vi "http 400 bad request.vi"(11 "application request in":T4) -> (3 "application request out":T1)   [LabVIEW 2016, in "Basic HTTP server.lvclass"]
uses:
  Basic HTTP server.lvclass
  http request.ctl
  http method.ctl
  http header data.ctl
  http response.ctl
  http response packet type.ctl
  headers/http headers.lvlib
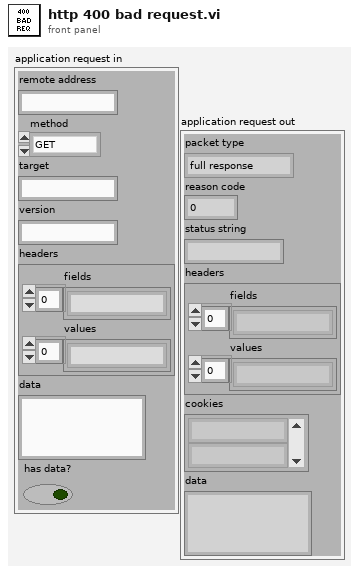
[diagram p1: front panel]
types:
  T1 = typedef "Basic HTTP server.lvclass/http response.ctl" = cluster{"packet type":T2, "reason code":u16, "status string":string, "headers":T3, "cookies":string[], "data":string}
  T2 = typedef "Basic HTTP server.lvclass/http response packet type.ctl" = enum16{"full response", "header only", "data only", "last data"}
  T3 = typedef "http headers.lvlib/http header data.ctl" = cluster{"fields":string[], "values":string[]}
  T4 = typedef "Basic HTTP server.lvclass/http request.ctl" = cluster{"remote address":string, "method":T5, "target":string, "version":string, "headers":T3, "data":string, "has data?":bool}
  T5 = typedef "Basic HTTP server.lvclass/http method.ctl" = enum16{"GET", "POST", "PUT", "DELETE", "HEAD", "OPTIONS", "upgrade"}
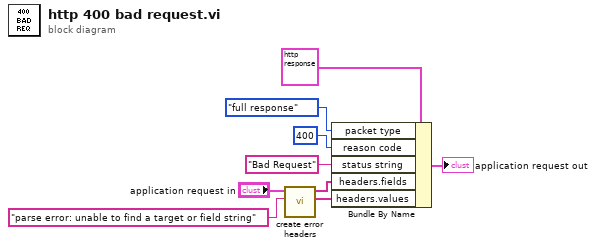
[diagram p0: block diagram]
diagram:
  n1 = call "create error headers.vi"("custom error reason"="parse error: unable to find a target or field string" ("name"), "application request in"="application request in") -> ("values"=w2:string[], "fields"=w1:string[])  [unwired: 8 in]
  n2 = Bundle By Name(cluster=T1 {"packet type"=enum."full response", "reason code"=0, "status string"="", "headers"={"fields"=[], "values"=[]}, "cookies"=[], "data"=""} ("application request"), "packet type"=http_response_packet_type."full response", "reason code"=u16 400, "status string"="Bad Request", "headers.fields"=w1, "headers.values"=w2) -> (→"application request out":T1)
